vi "Remote control temp ACCEL ver 2.vi"() -> ()   [LabVIEW 2018]
panel:
  out "Speed":T1
  out "ServoGrip":bool
  out "Directions":string
  in  "stop":bool
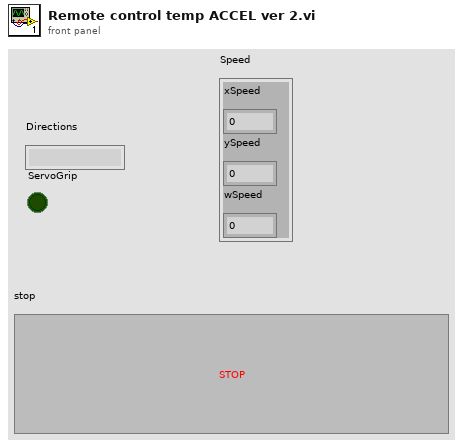
[diagram p1: front panel]
types:
  T1 = cluster{"xSpeed":dbl, "ySpeed":dbl, "wSpeed":dbl}
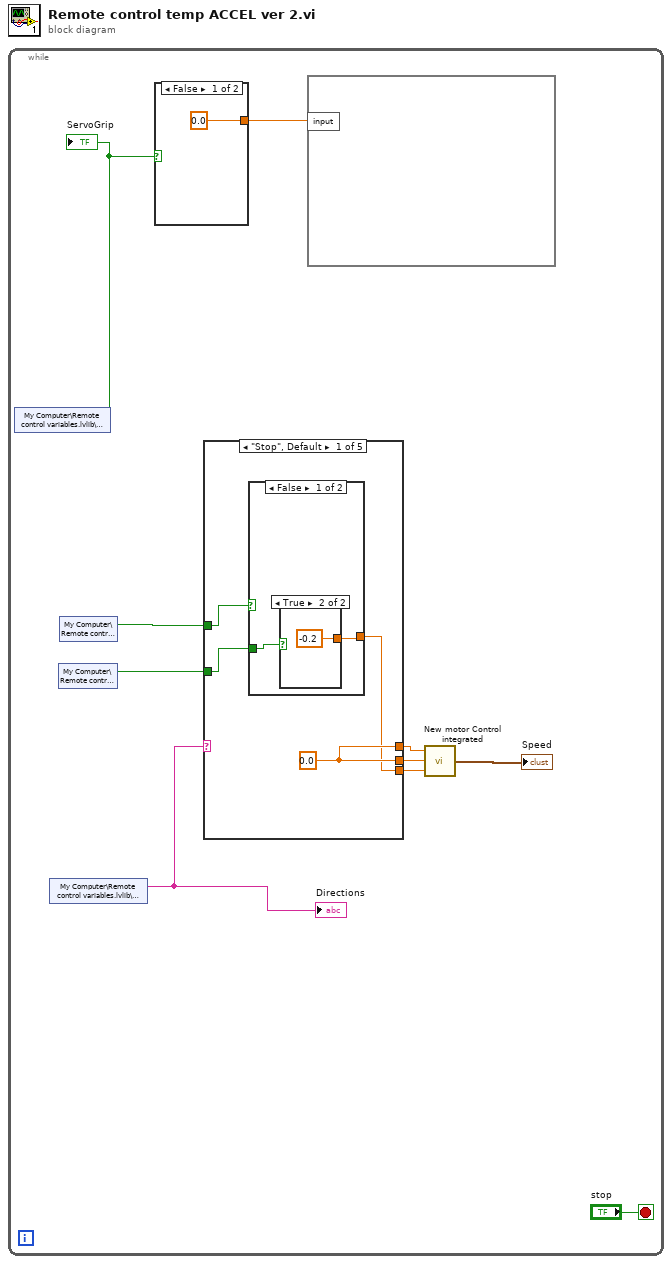
[diagram p0: block diagram]
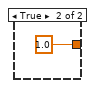
[diagram p2: hidden frame]
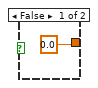
[diagram p3: hidden frame]
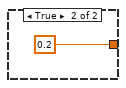
[diagram p4: hidden frame]
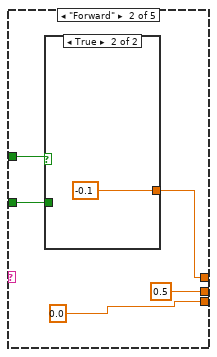
[diagram p5: hidden frame]
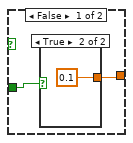
[diagram p6: hidden frame]
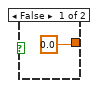
[diagram p7: hidden frame]
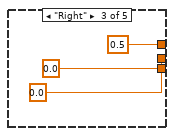
[diagram p8: hidden frame]
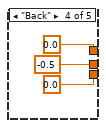
[diagram p9: hidden frame]
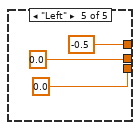
[diagram p10: hidden frame]
diagram:
  n1 = while {
    stop <- "stop" stop-if-true
    n2 = shared-variable "My Computer\\Remote control variables.lvlib\\ServoGrip"() -> (w6:bool)  [unwired: 1 in, 1 out]
    "ServoGrip" <- w6
    n3 = shared-variable "My Computer\\Remote control variables.lvlib\\Directions"() -> (w9:string)  [unwired: 1 in, 1 out]
    "Directions" <- w9
    n4 = shared-variable "My Computer\\Remote control variables.lvlib\\RB"() -> (w7:bool)  [unwired: 1 in, 1 out]
    n5 = shared-variable "My Computer\\Remote control variables.lvlib\\LB"() -> (w8:bool)  [unwired: 1 in, 1 out]
    n6 = case shown="False" w6 {
      tunnel: [0.0 1.0] -> w5
      frame False {
      }
      frame True {
      }
    }
    n7 = case shown="\"Stop\", Default" w9 {
      tunnel: [w14 0.5 0.0 -0.5 0.0] -> w4
      tunnel: [w14 w23 0.5 0.0 -0.5] -> w3
      tunnel: [w13 0.0 0.0 0.0 0.0] -> w2
      tunnel: w8 -> [w16 w24 _ _ _]
      tunnel: w7 -> [w15 w22 _ _ _]
      frame "Stop", Default {
        w14 = 0.0
        n8 = case shown="False" w16 {
          tunnel: [w17 0.2] -> w13
          tunnel: w15 -> [w18 _]
          frame False {
            n9 = case shown="True" w18 {
              tunnel: [0.0 -0.2] -> w17
              frame False {
              }
              frame True {
              }
            }
          }
          frame True {
          }
        }
      }
      frame "Forward" {
        n10 = case shown="True" w24 {
          tunnel: [w27 -0.1] -> w23
          tunnel: w22 -> [w28 _]
          frame False {
            n11 = case shown="True" w28 {
              tunnel: [0.0 0.1] -> w27
              frame False {
              }
              frame True {
              }
            }
          }
          frame True {
          }
        }
      }
      frame "Right" {
      }
      frame "Back" {
      }
      frame "Left" {
      }
    }
    n12 = formula code=""("input"=w5) -> ()
    n13 = call "New motor Control integrated.vi"("wTargetSpeed"=w2, "yTargetSpeed"=w4, "xTargetSpeed"=w3) -> ("Speed"=→"Speed":T1)
  }
